vi "Get_ADAM_averages_server.vi"(5 "No of averages":i32=1, 6 "All Active Channels":bool, 7 "End time":dbl, 8 "Start time":dbl, 9 "Clients time":dbl, 10 "ADAM Ch Names":string[](array[string])) -> (0 "DBL values":dbl[][](array[numeric]) format="%.2f", 1 "Values":string[][](array[string]), 2 "Comments":string[](array[string]), 3 "Titles":string[](array[string]), 4 "Times":dbl[](array[numeric]) format="%.2f")   [LabVIEW 2010]
uses:
  ADAM_Global.vi
  Sub VI's/Logged_Data_real_Global.vi
  Sub VI's/Channel_Description_Global.vi
panel:
  out "Client leads me by:":dbl
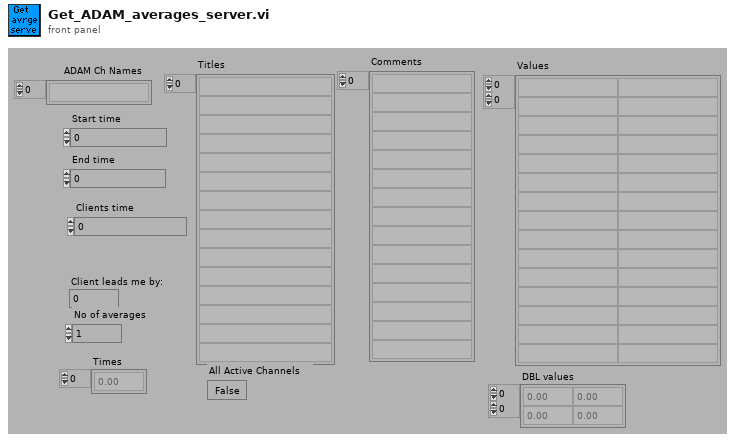
[diagram p1: front panel]
types:
  T1 = typedef "Ch_description_ADAM.ctl" = cluster{"Ch Name":string, "Type":T2, "Function":T3, "Ch State":T4, "Calibration type":T5, "A":dbl, "B":dbl, "C":dbl, "D":dbl, "Comments":string, "Address":T6, "String":string, "Duty":u16}
  T2 = typedef "Module_type_ADAM.ctl" = enum16{"4011", "4012", "4013", "4014", "4016", "4017", "4018", "4021", "4050", "4052", "4053", "4060", "4080", "5000", "5017", "5018", "5024", "5051", "5056", "5060", "6060", "Tracker", "WEST", "GILL", "JEM", "VICI", "Vaisala", "DRUCK", "Run VI Named:", "IR2100", "PPT", "Comparator", "VIRTUAL", "Hold Value", "Read A", "Read Ch", "Coded", "Client Info", "Web Client", "X10", "Test"}
  T3 = typedef "Function_ADAM.ctl" = enum16{"Analogue Input", "Digital Input", "Event counter", "Event rate", "Analogue Output", "Digital Output", "Relay Output"}
  T4 = typedef "Channel_State.ctl" = enum16{"On", "Off", "Always On", "Always Off"}
  T5 = typedef "Calib_type_ADAM.ctl" = enum16{"Raw", "Bx + A", "Cx^2 + Bx + A", "Dx^3 + Cx^2 + Bx + A", "In Band", "Hi-Tec Q", "Hi-Tec M_dot", "Text"}
  T6 = typedef "Address.ctl" = cluster{"Main":i32, "Ch.":i32, "Sub":i32, "Port Name":string}
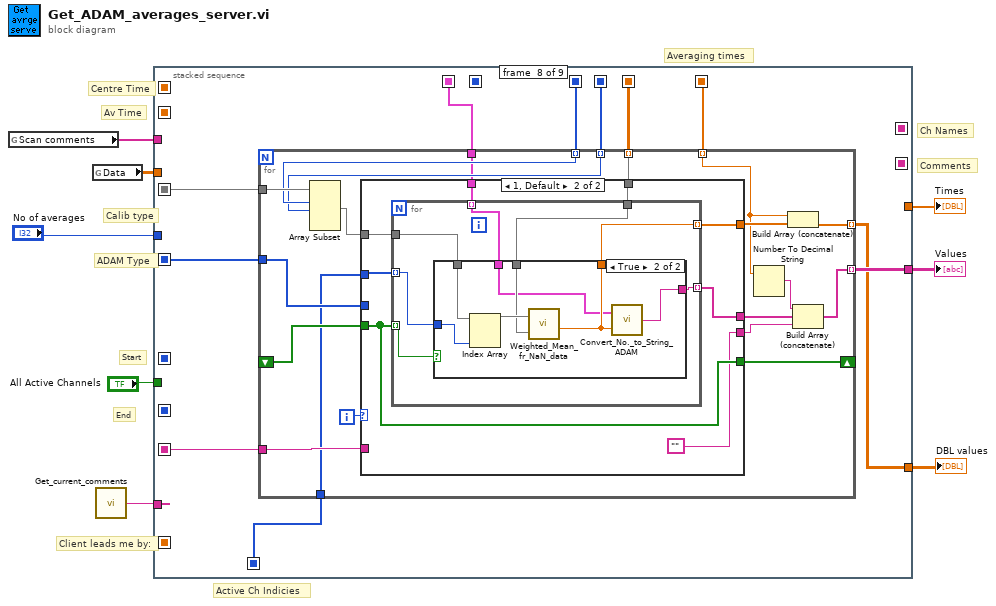
[diagram p0: block diagram]
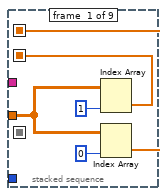
[diagram p2: hidden frame]
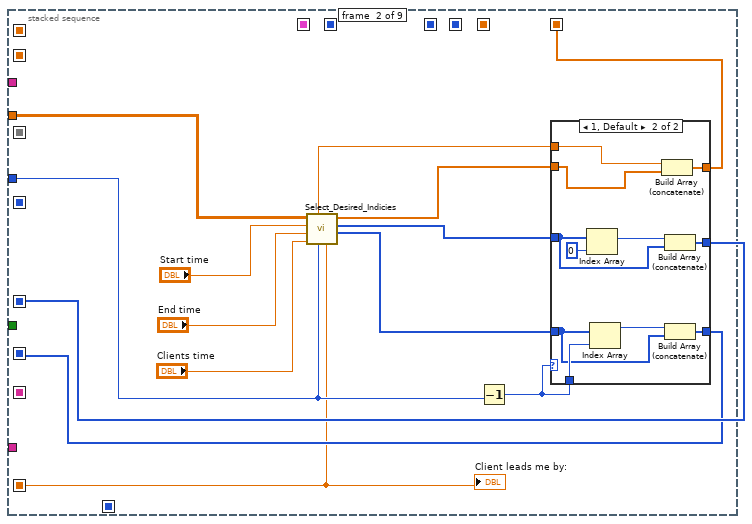
[diagram p3: hidden frame]
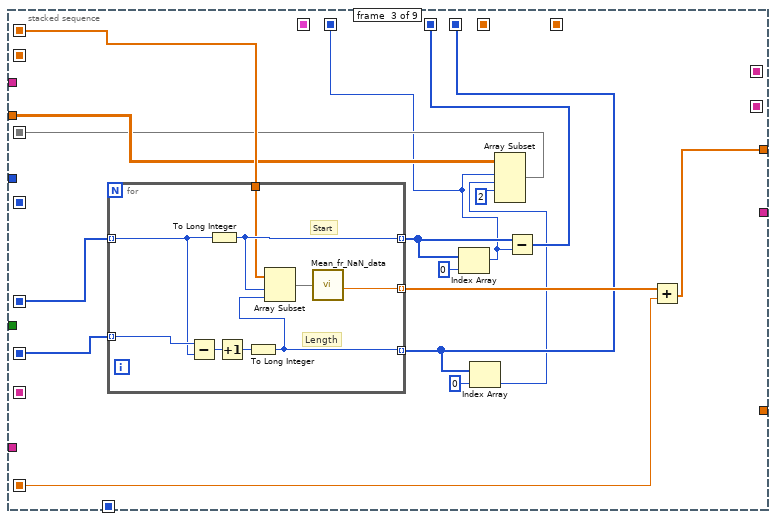
[diagram p5: hidden frame]
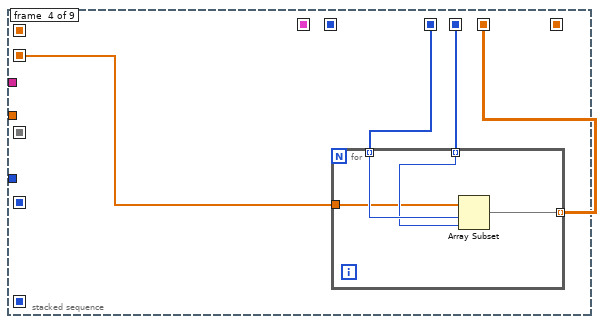
[diagram p6: hidden frame]
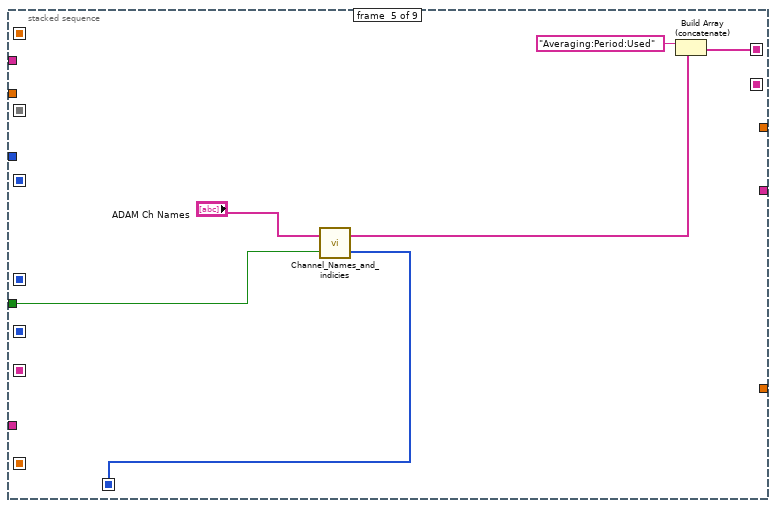
[diagram p7: hidden frame]
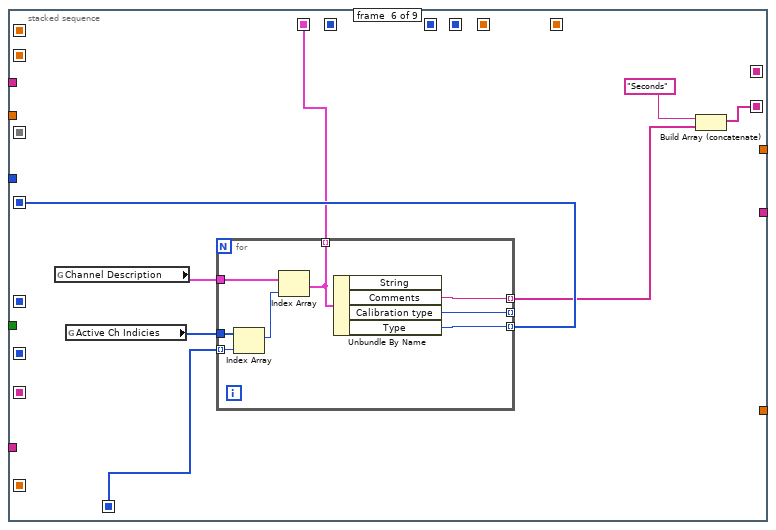
[diagram p8: hidden frame]
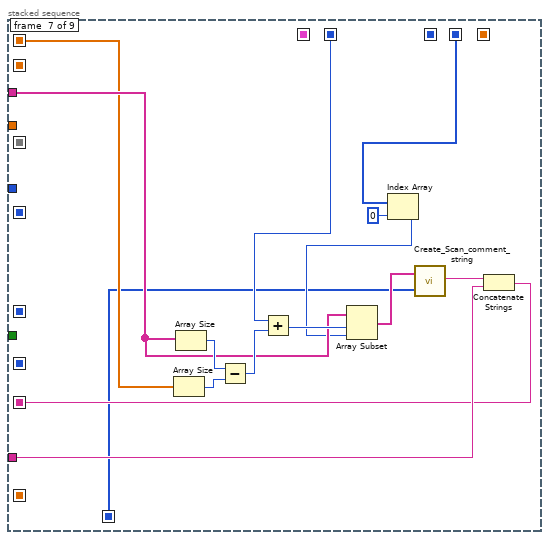
[diagram p9: hidden frame]
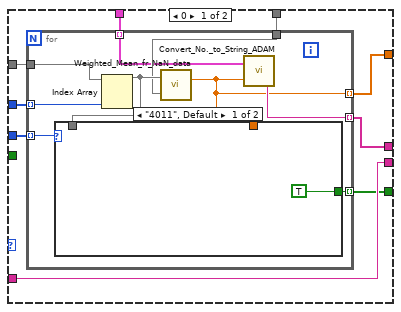
[diagram p10: hidden frame]
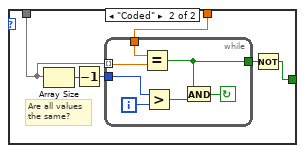
[diagram p11: hidden frame]
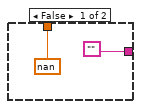
[diagram p12: hidden frame]
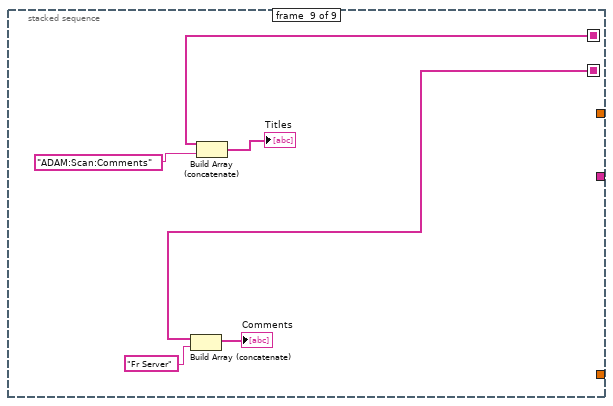
[diagram p13: hidden frame]
diagram:
  # "Averaging times"
  # "End"
  # "Start"
  # "Av Time"
  # "Centre Time"
  # "Active Ch Indicies"
  # "ADAM Type"
  # "Calib type"
  # "Ch Names"
  # "Comments"
  # "Client leads me by:"
  n1 = global read "ADAM_Global.vi" "Scan comments"() -> (w6:string[])
  n2 = global read "Logged_Data_real_Global.vi" "Data"() -> (w1:dbl[][])
  n3 = call "Get_current_comments.vi"() -> ("Comment"=w7:string)
  n4 = stacked-sequence {
    seq-local: [_ _ w48 _ _ _ _ _ _] -> [_ _ _ w69 _ _ w102 w121 _]
    seq-local: [_ _ w50 _ _ _ _ _ _] -> [_ _ _ w70 _ _ _ w122 _]
    seq-local: [_ _ w46 _ _ _ _ _ _] -> [_ _ _ _ _ _ _ w120 _]
    seq-local: [_ w27 _ _ _ _ _ _ _] -> [_ _ w55 _ _ _ _ _ _]
    seq-local: [_ w26 _ _ _ _ _ _ _] -> [_ _ w54 _ _ _ _ _ _]
    seq-local: [w11 _ _ _ _ _ _ _ _] -> [_ _ w53 _ _ _ w105 _ _]
    seq-local: [_ _ w45 _ _ _ _ _ _] -> [_ _ _ _ _ _ w104 _ _]
    seq-local: [_ _ _ _ _ _ w98 _ _] -> [_ _ _ _ _ _ _ w118 _]
    seq-local: [_ _ _ _ _ w88 _ _ _] -> [_ _ _ _ _ _ _ w117 _]
    seq-local: [_ w16 _ _ _ _ _ _ _] -> [_ _ _ _ _ _ _ w116 _]
    seq-local: [_ _ _ w68 _ _ _ _ _] -> [_ _ _ _ _ _ _ w115 _]
    seq-local: [_ _ _ _ w79 _ _ _ _] -> [_ _ _ _ _ _ _ _ w199]
    seq-local: [_ _ _ _ _ w85 _ _ _] -> [_ _ _ _ _ _ _ _ w198]
    seq-local: [_ w17 _ _ _ _ _ _ _] -> [_ _ w42 _ _ _ _ _ _]
    seq-local: [_ _ _ _ w76 _ _ _ _] -> [_ _ _ _ _ w83 w97 w113 _]
    seq-local: [w10 _ _ _ _ _ _ _ _] -> [_ _ _ w67 _ _ _ _ _]
    seq-local: [_ _ _ _ _ w81 _ _ _] -> [_ _ _ _ _ _ _ w112 _]
    tunnel: w1 -> [w9 w20 w47 _ _ _ _ _ _]
    tunnel: "No of averages" -> [_ w18 _ _ _ _ _ _ _]
    tunnel: [_ _ w56 _ _ _ _ _ _] -> w4
    tunnel: [_ _ _ _ _ _ _ w119 _] -> w5
    tunnel: [_ _ _ _ _ _ _ w114 _] -> w3
    tunnel: w6 -> [_ _ _ _ _ _ w106 _ _]
    tunnel: w7 -> [_ _ _ _ _ _ w99 _ _]
    tunnel: "All Active Channels" -> [_ _ _ _ w75 _ _ _ _]
    frame #0 {
      n5 = Index Array(array=w9, index (col)=1) -> (element=w10:dbl[])  [unwired: 1 in]
      n6 = Index Array(array=w9, index (col)=0) -> (element=w11:dbl[])  [unwired: 1 in]
    }
    frame #1 {
      n7 = call "Select_Desired_Indicies.vi"("No of averages"=w18, "Clients time"="Clients time", "End time"="End time", "Start time"="Start time", "Table values"=w20) -> ("End Integer"=w22:i32[], "Start integer"=w21:i32[], "Averaging Times"=w15:dbl[], "Client leads me by:"=w17:dbl, "Total Time"=w14:dbl)  [unwired: 1 out]
      "Client leads me by:" <- w17
      n8 = Decrement(x=w18) -> (x-1=w19:i32)
      n9 = case shown="1, Default" w19 {
        tunnel: w19 -> [_ w40]
        tunnel: w21 -> [w30 w38]
        tunnel: w22 -> [w29 w36]
        tunnel: [w30 w35] -> w27
        tunnel: [w29 w34] -> w26
        tunnel: [w28 w32] -> w16
        tunnel: w15 -> [w28 w33]
        tunnel: w14 -> [_ w31]
        frame 0 {
        }
        frame 1, Default {
          n10 = Index Array(array=w38, index=0 ("Index")) -> (element=w39:i32)
          n11 = Index Array(array=w36, index=w40) -> (element=w37:i32)
          n12 = Build Array (concatenate)(w31, w33) -> (w32:dbl[])
          n13 = Build Array (concatenate)(w39, w38) -> (w35:i32[])
          n14 = Build Array (concatenate)(w37, w36) -> (w34:i32[])
        }
      }
    }
    frame #2 {
      n15 = for {
        tunnel: [w64] -> w51 mode=indexing
        tunnel: [w63] -> w48 mode=indexing
        tunnel: [w61] -> w57 mode=indexing
        tunnel: w55 -> [w58] mode=indexing
        tunnel: w54 -> [w59] mode=indexing
        tunnel: w53 -> [w60]
        # "Length"
        # "Start"
        n16 = Subtract(x=w59, y=w58) -> (x-y=w65:i32)
        n17 = To Long Integer(number=w58) -> (32bit integer=w64:i32)
        n18 = Increment(x=w65) -> (x+1=w66:i32)
        n19 = To Long Integer(number=w66) -> (32bit integer=w63:i32)
        n20 = Array Subset(array=w60, index=w64, length=w63) -> (w62:dbl[])
        n21 = call "Mean_fr_NaN_data.vi"("Data"=w62) -> ("Mean value"=w61:dbl)
      }
      n22 = Index Array(array=w51, index=0 ("Index")) -> (element=w45:i32)
      n23 = Index Array(array=w48, index=0 ("Index")) -> (element=w44:i32)
      n24 = Array Subset(array=w47, index (row)=w45, length (row)=w44, index (col)=2 ("Array Index")) -> (w46:dbl[][])  [unwired: 1 in]
      n25 = Subtract(x=w51, y=w45) -> (x-y=w50:i32[])
      n26 = Add(x=w57, y=w42) -> (x+y=w56:dbl[])
    }
    frame #3 {
      n27 = for {
        tunnel: w70 -> [w74] mode=indexing
        tunnel: w69 -> [w73] mode=indexing
        tunnel: w67 -> [w72]
        tunnel: [w71] -> w68 mode=indexing
        n28 = Array Subset(array=w72, index=w74, length=w73) -> (w71:dbl[])
      }
    }
    frame #4 {
      n29 = call "Channel_Names_and_indicies.vi"("All Active Channels"=w75, "Desired Ch Names"="ADAM Ch Names") -> ("Indicies"=w76:i32[], "Active Ch names"=w77:string[])
      n30 = Build Array (concatenate)("Averaging:Period:Used" ("Input Element"), w77) -> (w79:string[])
    }
    frame #5 {
      n31 = global read "Channel_Description_Global.vi" "Channel Description"() -> (w82:T1[])
      n32 = global read "ADAM_Global.vi" "Active Ch Indicies"() -> (w84:i32[])
      n33 = for {
        tunnel: w82 -> [w96]
        tunnel: [w95] -> w86 mode=indexing
        tunnel: [w94] -> _ mode=indexing
        tunnel: [w93] -> w88 mode=indexing
        tunnel: w84 -> [w92]
        tunnel: w83 -> [w91] mode=indexing
        tunnel: [w89] -> w81 mode=indexing
        n34 = Index Array(array=w92, index=w91) -> (element=w90:i32)
        n35 = Index Array(array=w96, index=w90) -> (element=w89:T1)
        n36 = Unbundle By Name(w89) -> ("Comments"=w95:string, "Calibration type"=w94:T5, "Type"=w93:T2)  [unwired: 1 out]
      }
      n37 = Build Array (concatenate)("Seconds" ("Input Element"), w86) -> (w85:string[])
    }
    frame #6 {
      n38 = Array Size(array=w105) -> (size(s)=w109:i32)
      n39 = Array Size(array=w106) -> (size(s)=w108:i32)
      n40 = Subtract(x=w108, y=w109) -> (x-y=w110:i32)
      n41 = Add(x=w104, y=w110) -> (x+y=w111:i32)
      n42 = Index Array(array=w102, index=0 ("Index")) -> (element=w101:i32)
      n43 = Array Subset(array=w106, index=w111, length=w101) -> (w107:string[])
      n44 = call "Create_Scan_comment_string.vi"("Requested channels"=w97, "Scan comments"=w107) -> ("Comment string"=w100:string)
      n45 = Concatenate Strings(w100, w99) -> (w98:string)
    }
    frame #7 {
      n46 = for {
        tunnel: w122 -> [w137] mode=indexing
        tunnel: w121 -> [w136] mode=indexing
        tunnel: w120 -> [w141]
        tunnel: [w138] -> w119 mode=indexing
        tunnel: w118 -> [w133]
        tunnel: w117 -> [w135]
        shift-right: [w131] -> _
        shift-left: _ -> [w130]
        tunnel: w116 -> [w124] mode=indexing
        tunnel: w115 -> [w129] mode=indexing
        tunnel: w113 -> [w128]
        tunnel: [w125] -> w114 mode=indexing
        tunnel: w112 -> [w123]
        i -> [w134]
        n47 = Array Subset(array=w141, index (row)=w137, length (row)=w136) -> (w140:dbl[][])  [unwired: 2 in]
        n48 = case shown="1, Default" w134 {
          tunnel: w140 -> [w150 w181]
          tunnel: [w149 w180] -> w139
          tunnel: w135 -> [w147 _]
          tunnel: w133 -> [w148 _]
          tunnel: [w148 ""] -> w132
          tunnel: [w146 w179] -> w131
          tunnel: w130 -> [_ w179]
          tunnel: w129 -> [w145 w177]
          tunnel: w128 -> [w144 w175]
          tunnel: [w143 w176] -> w126
          tunnel: w123 -> [w142 w174]
          frame 0 {
            n49 = for {
              tunnel: w150 -> [w158]
              tunnel: [w159] -> w149 mode=indexing
              tunnel: w147 -> [w157] mode=indexing
              tunnel: [w155] -> w146 mode=indexing
              tunnel: w145 -> [w154]
              tunnel: w144 -> [w153] mode=indexing
              tunnel: [w152] -> w143 mode=indexing
              tunnel: w142 -> [w151] mode=indexing
              n50 = Index Array(array=w158, index (col)=w153) -> (element=w156:dbl[])  [unwired: 1 in]
              n51 = call "Weighted_Mean_fr_NaN_data.vi"("Weighting"=w154, "Data"=w156) -> ("Mean value"=w152:dbl)
              n52 = case shown="\"4011\", Default" w157 {
                tunnel: w156 -> [_ w164]
                tunnel: w152 -> [_ w163]
                tunnel: [TRUE w162] -> w155
                frame "4011", Default {
                }
                frame "Coded" {
                  # "Are all values the same?"
                  n53 = Array Size(array=w164) -> (size(s)=w165:i32)
                  n54 = Decrement(x=w165) -> (x-1=w166:i32)
                  n55 = while {
                    tunnel: w163 -> [w167]
                    tunnel: [w170] -> w161
                    tunnel: w164 -> [w169] mode=indexing
                    tunnel: w166 -> [w173]
                    i -> [w168]
                    stop <- w171 continue-if-true
                    n56 = Equal?(x=w167, y=w169) -> (x = y?=w170:bool)
                    n57 = Greater?(x=w173, y=w168) -> (0:w172:bool)
                    n58 = And(x=w170, y=w172) -> (x .and. y?=w171:bool)
                  }
                  n59 = Not(x=w161) -> (.not. x?=w162:bool)
                }
              }
              n60 = call "Convert_No._to_String_ADAM.vi"("Input number"=w152, "Ch Description"=w151) -> ("Output sting"=w159:string)
            }
          }
          frame 1, Default {
            n61 = for {
              tunnel: w181 -> [w187]
              tunnel: [w188] -> w180 mode=indexing
              tunnel: w179 -> [w186] mode=indexing
              tunnel: w177 -> [w185]
              tunnel: [w184] -> w176 mode=indexing
              tunnel: w175 -> [w183] mode=indexing
              tunnel: w174 -> [w182] mode=indexing
              n62 = case shown="True" w186 {
                tunnel: ["" w197] -> w188
                tunnel: w187 -> [_ w196]
                tunnel: w185 -> [_ w194]
                tunnel: [nan ("Mean value") w193] -> w184
                tunnel: w183 -> [_ w192]
                tunnel: w182 -> [_ w191]
                frame False {
                }
                frame True {
                  n63 = Index Array(array=w196, index (col)=w192) -> (element=w195:dbl[])  [unwired: 1 in]
                  n64 = call "Weighted_Mean_fr_NaN_data.vi"("Weighting"=w194, "Data"=w195) -> ("Mean value"=w193:dbl)
                  n65 = call "Convert_No._to_String_ADAM.vi"("Input number"=w193, "Ch Description"=w191) -> ("Output sting"=w197:string)
                }
              }
            }
          }
        }
        n66 = Number To Decimal String(number=w124) -> (decimal integer string=w127:string)  [unwired: 1 out]
        n67 = Build Array (concatenate)(w124, w126) -> (w125:dbl[])
        n68 = Build Array (concatenate)(w127, w139, w132) -> (w138:string[])
      }
    }
    frame #8 {
      n69 = Build Array (concatenate)(w198, "Fr Server" ("Comments")) -> (→"Comments":string[])
      n70 = Build Array (concatenate)(w199, "ADAM:Scan:Comments") -> (→"Titles":string[])
    }
  }
  "Values" <- w5
  "Times" <- w4
  "DBL values" <- w3
